vi "Voltage - Continuous Input.vi"() -> ()   [LabVIEW 2012]
doc: "该范例演示了如果使用DAQmx设备连续采集带缓冲的电压信号。\n\n关于如何连接信号至DAQ设备，请查看设备文档。"
uses:
  <vilib>/DAQmx/read.llb/DAQmx Read (Analog 1D Wfm NChan NSamp).vi
  <vilib>/DAQmx/create/channels.llb/DAQmx Create Channel (AI-Voltage-Basic).vi
  <vilib>/DAQmx/configure/timing.llb/DAQmx Timing (Sample Clock).vi
  <vilib>/DAQmx/configure/task.llb/DAQmx Configure Logging (TDMS).vi
  <vilib>/DAQmx/miscellaneous.llb/DAQmx Fill In Error Info.vi
  <resource>/objmgr/daqmx.rc
panel:
  in  "停止":bool
  out "波形图":waveform(dbl)[](graph)
  in  "TDMS文件路径":path
  in  "每个循环采样点":i32=1000
  in  "采样率":dbl=1000.0
  in  "采样时钟源":tag="OnboardClock"
  in  "接线端配置":i32(ring)=-1 items=["默认"=-1, "RSE"=10083, "NRSE"=10078, "差分"=10106, "伪差分"=12529]
  in  "最大电压":dbl=5.0
  in  "最小电压":dbl=-5.0
  in  "物理通道":tag="Dev1/ai0"
  out "实际采样率":dbl=1000.0 format="%0.2f"
  in  "记录模式":i32(ring)=10231 items=["关"=10231, "记录并读取"=15842]
  # "通道设置"
  # "采集数据"
  # "定时设置"
  # "记录设置"
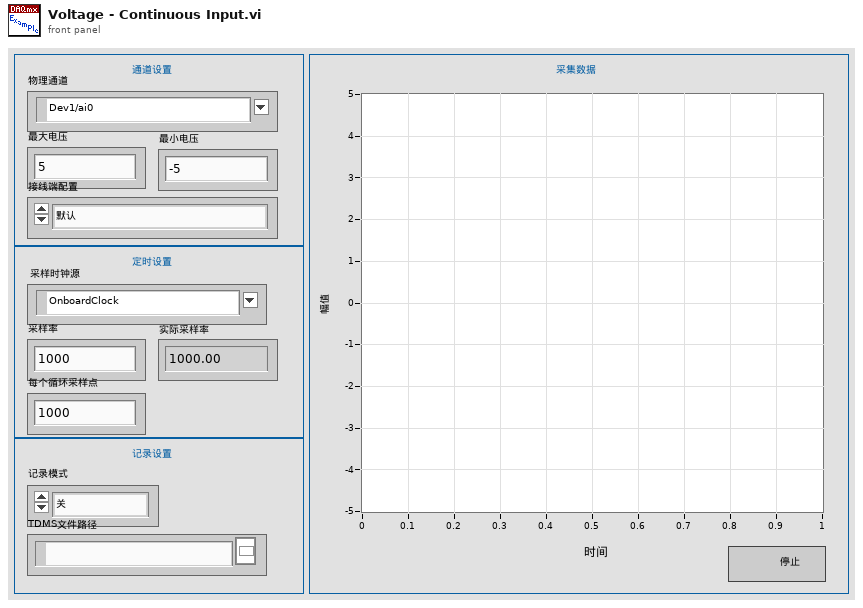
[diagram p1: front panel]
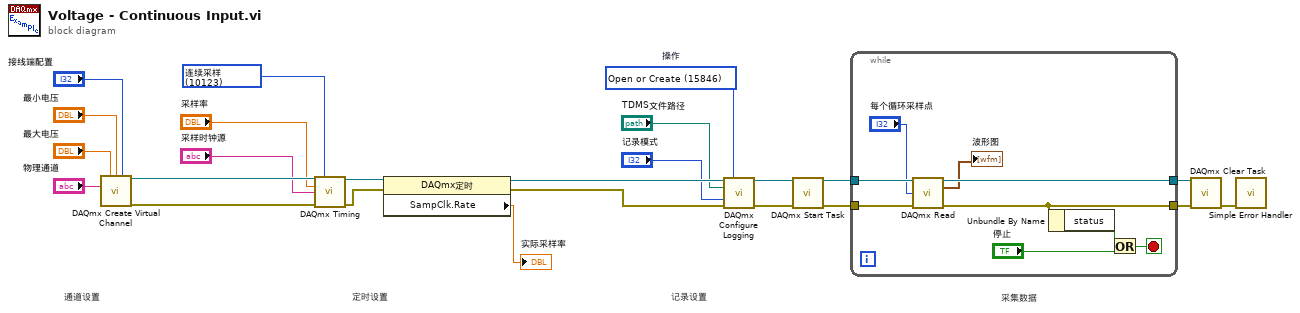
[diagram p0: block diagram]
diagram:
  w1 = 10123 items=["有限采样"=10178, "连续采样"=10123, "硬件定时单点"=12522] ("sample mode")
  w18 = 15846 items=["Open"=10437, "Open or Create"=15846, "Create or Replace"=15847, "Create"=15848]  # 操作
  # "采集数据"
  # "定时设置"
  # "通道设置"
  # "记录设置"
  n1 = call-poly <vilib>:"DAQmx Create Virtual Channel.vi"("maximum value"="最大电压", "minimum value"="最小电压", "input terminal configuration"="接线端配置", "physical channels"="物理通道") -> ("task out"=w21:refnum<k21>, "error out"=w22:errorcluster)  [unwired: 10 in]
  n2 = call-poly <vilib>:"DAQmx Timing.vi"("task/channels in"=w21, "sample mode"=w1, "rate"="采样率", "source"="采样时钟源", "error in"=w22) -> ("task out"=w24:refnum<k21>, "error out"=w23:errorcluster)  [unwired: 9 in]
  n3 = property on="属性节点" class="DAQmx定时"(reference=w24, error in=w23) -> (reference out=w20:refnum<k21>, error out=w19:errorcluster, "SampClk.Rate"=→"实际采样率":dbl)
  n4 = call-poly <vilib>:"DAQmx Configure Logging.vi"("task/channels in"=w20, "operation"=w18, "file path"="TDMS文件路径", "logging mode"="记录模式", "error in"=w19) -> ("task out"=w3:refnum<k21>, "error out"=w2:errorcluster)  [unwired: 9 in]
  n5 = call <vilib>:"DAQmx Start Task.vi"("task/channels in"=w3, "error in"=w2) -> ("task out"=w17:refnum<k21>, "error out"=w16:errorcluster)  [unwired: 12 in]
  n6 = while {
    tunnel: w17 -> [w33]
    tunnel: w16 -> [w32]
    tunnel: [w29] -> w14
    tunnel: [w30] -> w15
    stop <- w31 stop-if-true
    n7 = call-poly <vilib>:"DAQmx Read.vi"("task/channels in"=w33, "number of samples per channel"="每个循环采样点", "error in"=w32) -> ("task out"=w30:refnum<k21>, "data"=→"波形图":waveform(dbl)[], "error out"=w29:errorcluster)  [unwired: 10 in]
    n8 = Unbundle By Name ("按名称解除捆绑")(w29) -> ("status"=w28:bool)
    n9 = Or ("或")(x=w28, y="停止") -> (x .or. y?=w31:bool)
  }
  n10 = call <vilib>:"DAQmx Clear Task.vi"("task in"=w15, "error in"=w14) -> ("error out"=w13:errorcluster)  [unwired: 13 in]
  n11 = call <vilib>:"Simple Error Handler.vi"("error in (no error)"=w13) -> ()  [unwired: 4 in, 5 out]
